vi "Compute Destination Endpoints.vi"(8 "error in":errorcluster, 9 "endpoints":string[](array[string]), 10 "source endpoint":string, 11 "slsc switch session in":T1) -> (0 "error out":errorcluster, 2 "possible destinations":string[](array[string]), 3 "slsc switch session out":T1)   [LabVIEW 2017, in "SLSC Switch Scripting.lvlib"]
uses:
  SLSC Switch Scripting.lvlib
  <vilib>/userdefined/High Color/SLSC_Switch/nislscslSession.ctl
  <vilib>/SLSC_Switch/Path Capability.ctl
  <vilib>/SLSC_Switch/SLSC Switch.lvlib
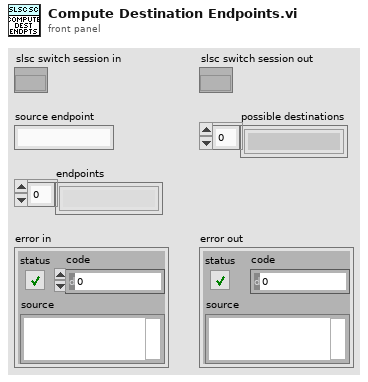
[diagram p1: front panel]
types:
  T1 = typedef "nislscslSession.ctl" = refnum<k20>
  T2 = typedef "SLSC Switch.lvlib/Path Capability.ctl" = i32
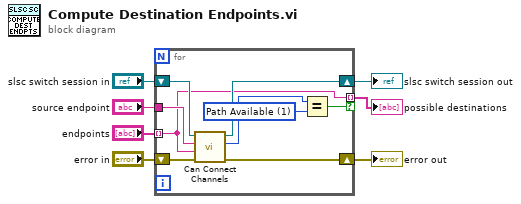
[diagram p0: block diagram]
diagram:
  n1 = for {
    tunnel: "endpoints" -> [w9] mode=indexing
    shift-right: [w15] -> w3
    shift-left: "error in" -> [w16]
    shift-right: [w13] -> w5
    shift-left: "slsc switch session in" -> [w14]
    tunnel: "source endpoint" -> [w12]
    tunnel: [w9] -> w7 mode=indexing if=w8
    w10 = T2 1 items=["Path Available"=1, "Path Exists"=2, "Path Unsupported"=3, "Resource in Use"=4, "Source Conflict"=5, "Channel Not Available"=6] ("y")
    n2 = call <vilib>:"Can Connect Channels.vi"("error in (no error)"=w16, "channel 2"=w9, "channel 1"=w12, "session in"=w14) -> ("error out"=w15:errorcluster, "path capability"=w11:T2, "session out"=w13:T1)  [unwired: 5 in]
    n3 = Equal?(x=w11, y=w10) -> (x = y?=w8:bool)
  }
  "possible destinations" <- w7
  "slsc switch session out" <- w5
  "error out" <- w3
